vi "Write TIFF Metadata General.vi"(8 "error in (no error)":errorcluster, 10 "Destination Image Path":path=path "C:/Users/Sebastien/Desktop/TIFF/data_000000_Metadata.tif", 11 "Source File Image Path":path=path "C:/Users/Sebastien/Desktop/TIFF/data_000000.tif") -> (0 "Error Out":errorcluster)   [LabVIEW 2025]
doc: "This software was created to prototype writing metadata to a TIFF file with a single image.\n\n<B>Usage:</B> This software is free to use, copy or plagiariaze. It is provided \"as-is\", and no technical support will be provided. The copyright is retained by NASA Marshall Space Flight Center.\n\n<B>Testing:</B> This software was tested by A) verifying that operations were completed successfully using LabVIEW 2009 on Windows XP, .NET version 4.0 and B) Windows Vista Microsoft Office Picture Manager was able to read and display the output file and C) Windows Vista Windows Photo Gallery was able to read and display the output file and the Description and D) Adobe Photoshop for Macintosh was able to correctly load and display the image and all the metadata.\n\n<B>Note:</B> This software requires .NET version 4.0\n\n<B>Warning:</B> This software will overwrite the destination file if it exists.\n\nThis software originally developed by:\nDerek Mayer\nBAE Systems - Technology Solutions & Services\n308 Voyager Way\nHuntsville, AL 35806\n(256) 890-8000\nwww.mevatec.com\nwww.baesystems.com/TSS\nSeptember 2010"
uses:
  System.Drawing
panel:
  out "Metadata OUT":T1(array[cluster])
  out "Metadata":T2
  in  "Description":string="Embryo - GFP-Septin - RFP-Myosin"
  in  "User":T3(ring)
  # "https://forums.ni.com/t5/LabVIEW/How-do-I-add-meta-tag-data-to-a-TIF-image-file/td-p/1221780"
  # "https://exiv2.org/tags.html"
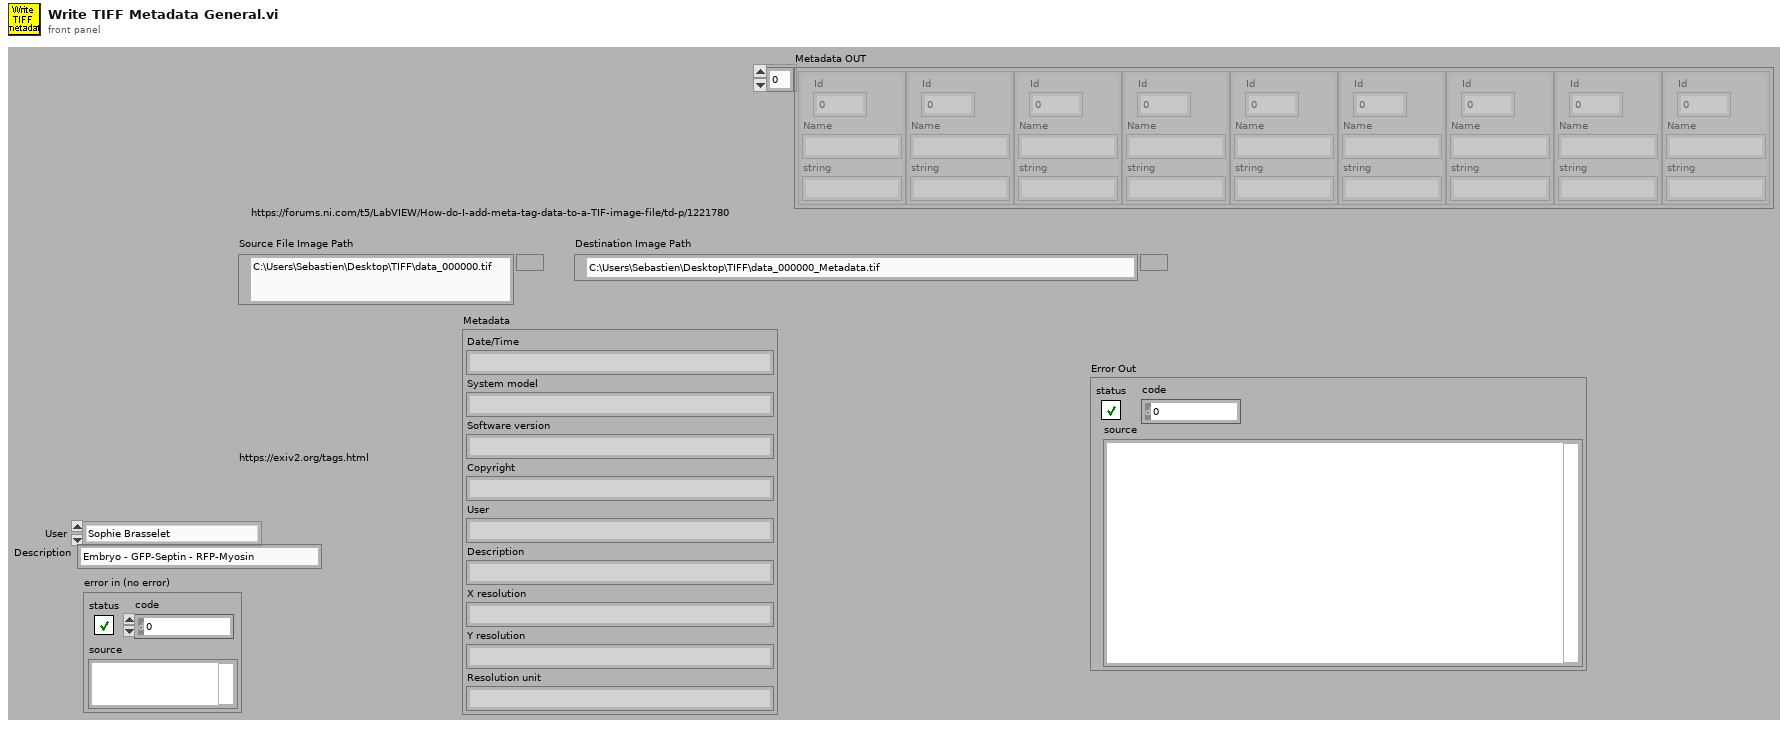
[diagram p1: front panel]
types:
  T1 = cluster{"Id":i32, "Name":string, "string":string}[]
  T2 = cluster{"Date/Time":string, "System model":string, "Software version":string, "Copyright":string, "User":string, "Description":string, "X resolution":string, "Y resolution":string, "Resolution unit":string}
  T3 = enum16{"Sophie Brasselet", "Jean-Jacques Honorine", "Sébastien Mailfert", "Manos Mavrakis"}
  T4 = cluster{"Error":errorcluster, "Source Filestream":refnum<k24>, "TIFF Decoder":refnum<k24>, "TIFF Frames":refnum<k24>, "get_Item":refnum<k24>, "Bitmap Metadata":refnum<k24>, "New Encoder":refnum<k24>}
  T5 = cluster{"ID":i32, "Name":string, "Notes":string}[]
  T6 = cluster{"Id":i32, "Name":string, "string":string}
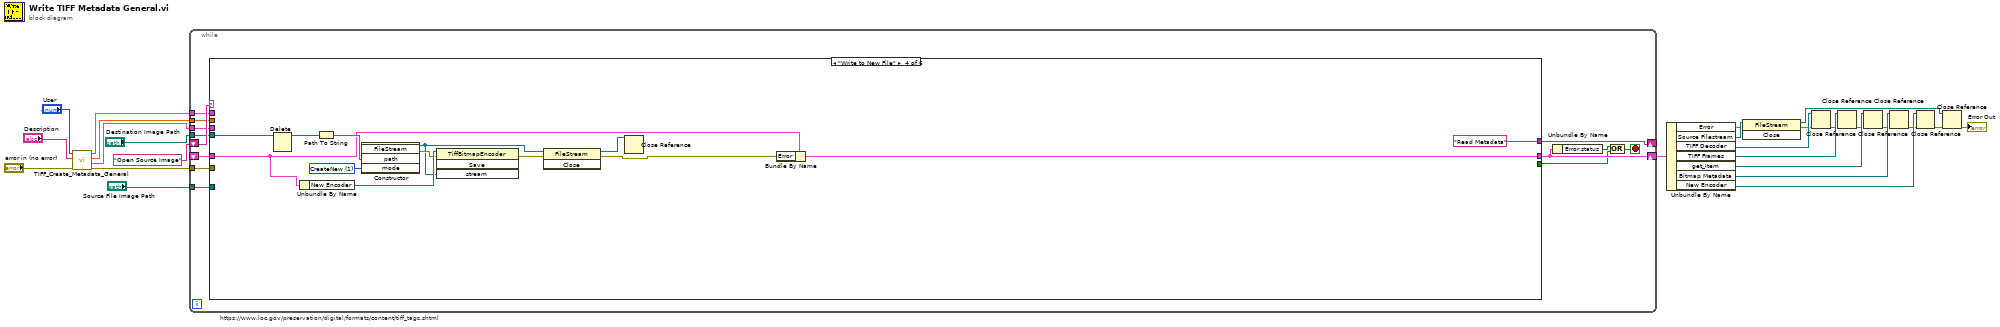
[diagram p0: block diagram]
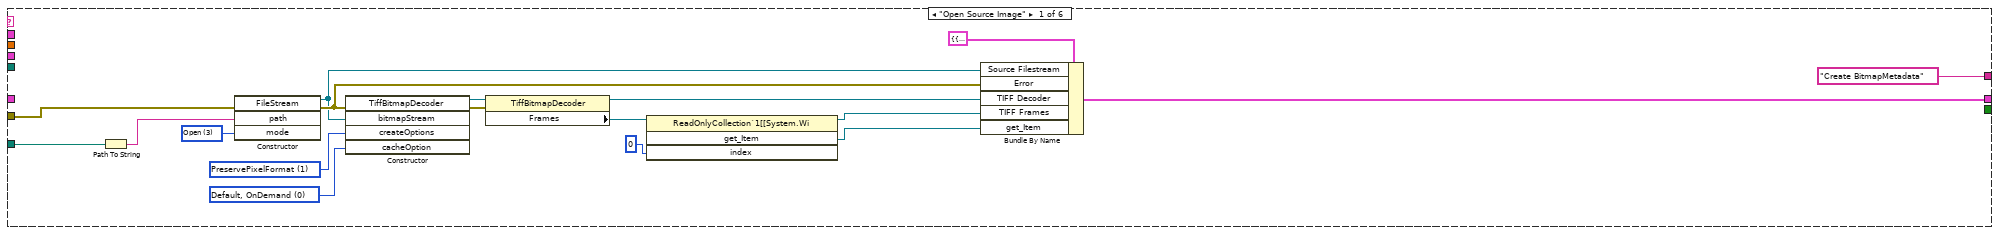
[diagram p2: hidden frame]
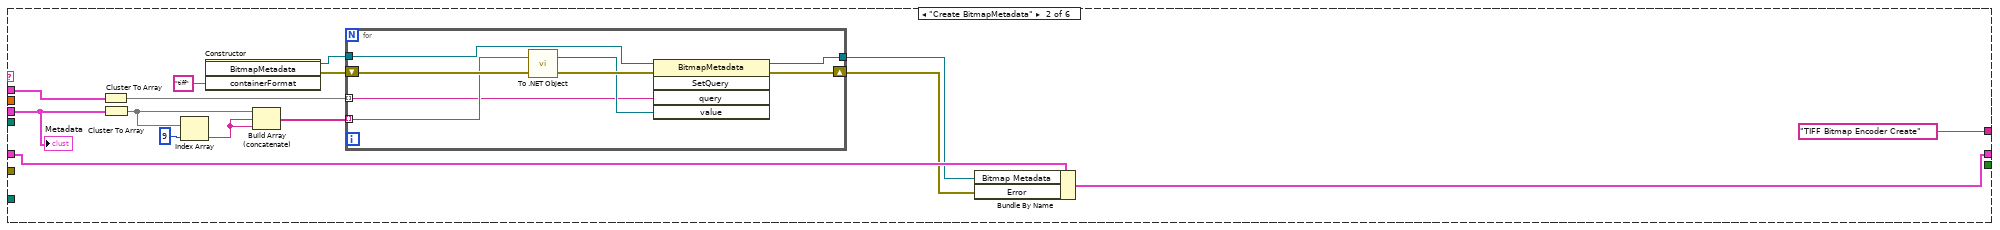
[diagram p3: hidden frame]
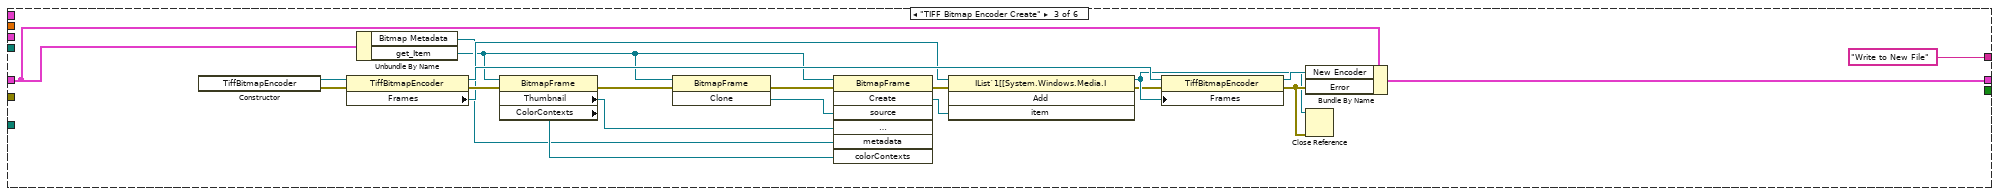
[diagram p4: hidden frame]
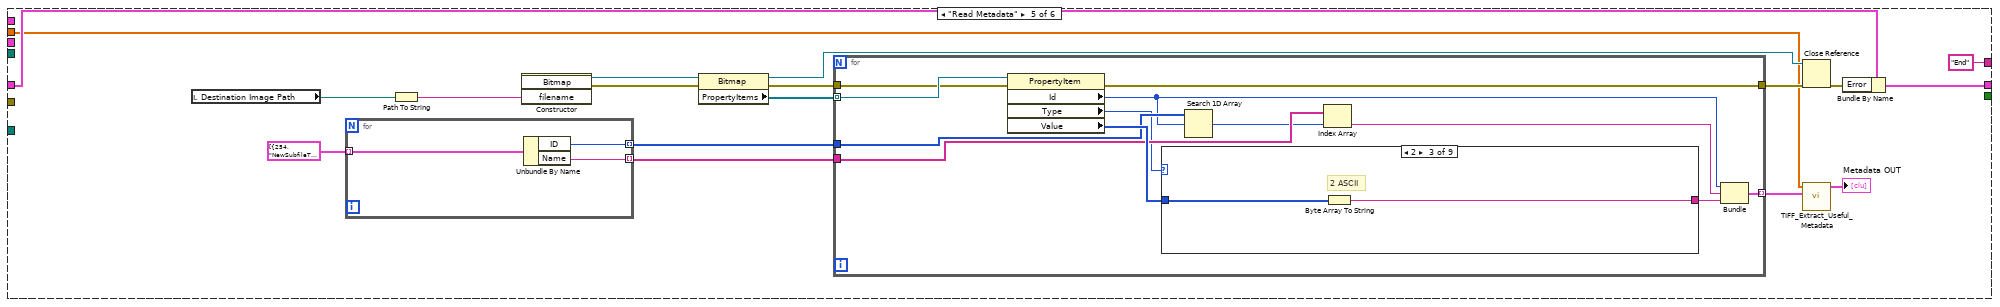
[diagram p5: hidden frame]
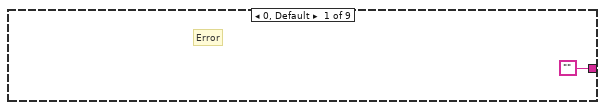
[diagram p6: hidden frame]
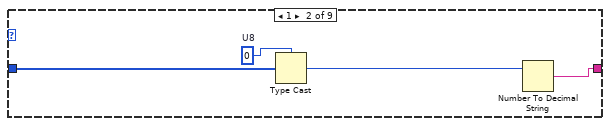
[diagram p7: hidden frame]
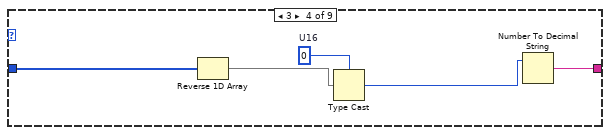
[diagram p8: hidden frame]
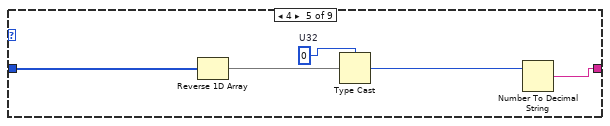
[diagram p9: hidden frame]
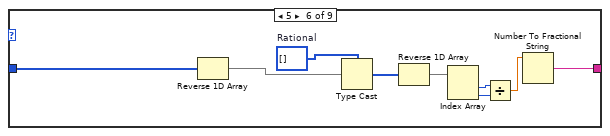
[diagram p10: hidden frame]
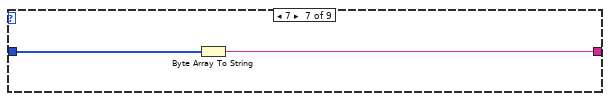
[diagram p11: hidden frame]
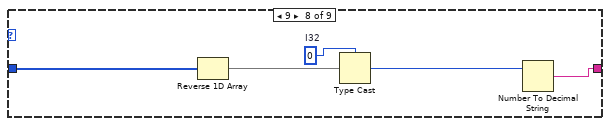
[diagram p12: hidden frame]
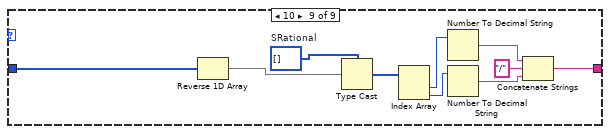
[diagram p13: hidden frame]
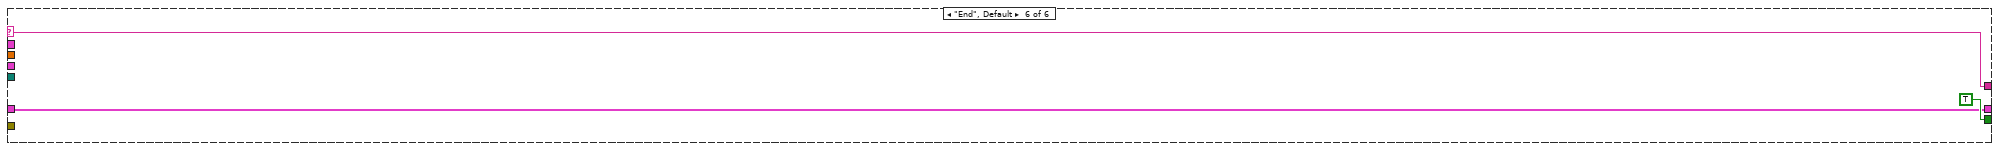
[diagram p14: hidden frame]
diagram:
  # "https://www.loc.gov/preservation/digital/formats/content/tiff_tags.shtml"
  n1 = call "TIFF_Create_Metadata_General.vi"("error in (no error)"="error in (no error)", "Description"="Description", "User"="User") -> ("error out"=w4:errorcluster, "Metadata OUT"=w2:T2, "Tag IDs"=w1:dbl[], "Taggs"=w3:T2)  [unwired: 5 in]
  n2 = while {
    shift-right: [w32] -> _
    shift-left: "Open Source Image" -> [w39]
    tunnel: "Source File Image Path" -> [w38]
    shift-right: [w37] -> w24
    shift-left: _ -> [w33]
    tunnel: "Destination Image Path" -> [w31]
    tunnel: w4 -> [w30]
    tunnel: w2 -> [w29]
    tunnel: w3 -> [w28]
    tunnel: w1 -> [w27]
    stop <- w34 stop-if-true
    n3 = case shown="\"Write to New File\"" w39 {
      selector: w39 -> [_ _ _ _ _ w191]
      tunnel: [_ _ _ _ _ TRUE] -> w36
      tunnel: w38 -> [w57 _ _ _ _ _]
      tunnel: [w53 w71 w101 w104 w119 w192] -> w37
      tunnel: w33 -> [_ w70 w98 w105 w120 w192]
      tunnel: ["Create BitmapMetadata" "TIFF Bitmap Encoder Create" "Write to New File" "Read Metadata" "End" w191] -> w32
      tunnel: w31 -> [_ _ _ w102 _ _]
      tunnel: w30 -> [w40 _ _ _ _ _]
      tunnel: w29 -> [_ w59 _ _ _ _]
      tunnel: w28 -> [_ w58 _ _ _ _]
      tunnel: w27 -> [_ _ _ _ w115 _]
      frame "Open Source Image" {
        w51 = 0 items=["Default, OnDemand", "OnLoad", "None"] ("cacheOption")
        w52 = 1 items=["None"=0, "PreservePixelFormat"=1, "DelayCreation"=2, "IgnoreColorProfile"=4, "IgnoreImageCache"=8] ("createOptions")
        w55 = 3 items=["CreateNew"=1, "Create"=2, "Open"=3, "OpenOrCreate"=4, "Truncate"=5, "Append"=6] ("mode")
        n4 = Path To String(path=w57) -> (string=w56:string)
        n5 = constructor class="FileStream"(error in=w40, "path"=w56, "mode"=w55) -> (reference out=w45:refnum<k24>, error out=w50:errorcluster)  [unwired: 2 in, 3 out]
        n6 = constructor class="TiffBitmapDecoder"(error in=w50, "bitmapStream"=w45, "createOptions"=w52, "cacheOption"=w51) -> (reference out=w48:refnum<k24>, error out=w49:errorcluster)  [unwired: 2 in, 4 out]
        n7 = property class="TiffBitmapDecoder"(reference=w48, error in=w49) -> (reference out=w44:refnum<k24>, "Frames"=w47:refnum<k24>)  [unwired: 1 out]
        n8 = invoke class="ReadOnlyCollection`1[[System.Wi" method="get_Item"(reference=w47, "index"=0) -> (reference out=w43:refnum<k24>, "get_Item"=w42:refnum<k24>)  [unwired: 2 in, 2 out]
        n9 = Bundle By Name(cluster=T4 {"Error"={"status"=FALSE, "code"=0, "source"=""}, "Source Filestream"=refnum, "TIFF Decoder"=refnum, "TIFF Frames"=refnum, "get_Item"=refnum, "Bitmap Metadata"=refnum, "New Encoder"=refnum}, "Source Filestream"=w45, "Error"=w50, "TIFF Decoder"=w44, "TIFF Frames"=w43, "get_Item"=w42) -> (w53:T4)
      }
      frame "Create BitmapMetadata" {
        n10 = Cluster To Array(cluster=w58) -> (array=w60:string[])
        n11 = Cluster To Array(cluster=w59) -> (array=w63:string[])
        n12 = Index Array(array=w63, index=9) -> (element=w64:string)
        n13 = constructor class="BitmapMetadata"("containerFormat"="tiff") -> (reference out=w69:refnum<k24>, error out=w68:errorcluster)  [unwired: 3 in, 2 out]
        n14 = Build Array (concatenate)(w63, w64, w64) -> (w62:string[])
        n15 = for {
          tunnel: [w77] -> w61
          tunnel: w69 -> [w74]
          shift-right: [w75] -> w66
          shift-left: w68 -> [w80]
          tunnel: w60 -> [w73] mode=indexing
          tunnel: w62 -> [w76] mode=indexing
          n16 = call <vilib>:"To .NET Object.vi"("error in (no error)"=w80, "anything"=w76) -> ("error out"=w79:errorcluster, ".NET object"=w78:refnum<k24>)
          n17 = invoke class="BitmapMetadata" method="SetQuery"(reference=w74, error in=w79, "query"=w73, "value"=w78) -> (reference out=w77:refnum<k24>, error out=w75:errorcluster)  [unwired: 1 in, 3 out]
        }
        n18 = Bundle By Name(cluster=w70, "Bitmap Metadata"=w61, "Error"=w66) -> (w71:T4)
        "Metadata" <- w59
      }
      frame "TIFF Bitmap Encoder Create" {
        n19 = constructor class="TiffBitmapEncoder"() -> (reference out=w90:refnum<k24>, error out=w99:errorcluster)  [unwired: 3 in, 1 out]
        n20 = property class="TiffBitmapEncoder"(reference=w90, error in=w99) -> (reference out=w94:refnum<k24>, error out=w93:errorcluster, "Frames"=w89:refnum<k24>)
        n21 = Unbundle By Name(w98) -> ("Bitmap Metadata"=w85:refnum<k24>, "get_Item"=w83:refnum<k24>)
        n22 = property class="BitmapFrame"(reference=w83, error in=w93) -> (error out=w95:errorcluster, "Thumbnail"=w87:refnum<k24>, "ColorContexts"=w88:refnum<k24>)  [unwired: 1 out]
        n23 = invoke class="BitmapFrame" method="Clone"(reference=w83, error in=w95) -> (error out=w82:errorcluster, "Clone"=w86:refnum<k24>)  [unwired: 1 in, 1 out]
        n24 = invoke class="BitmapFrame" method="Create"(reference=w83, error in=w82, "source"=w86, "thumbnail"=w87, "metadata"=w85, "colorContexts"=w88) -> (error out=w81:errorcluster, "Create"=w84:refnum<k24>)  [unwired: 1 in, 5 out]
        n25 = invoke class="IList`1[[System.Windows.Media.I" method="Add"(reference=w89, error in=w81, "item"=w84) -> (reference out=w92:refnum<k24>, error out=w91:errorcluster)  [unwired: 1 in, 2 out]
        n26 = property class="TiffBitmapEncoder"(reference=w94, error in=w91, "Frames"=w92) -> (reference out=w97:refnum<k24>, error out=w96:errorcluster)
        n27 = Bundle By Name(cluster=w98, "New Encoder"=w97, "Error"=w96) -> (w101:T4)
        n28 = Close Reference(reference=w92, error in (no error)=w96) -> ()  [unwired: 1 out]
      }
      frame "Write to New File" {
        w111 = 1 items=["CreateNew"=1, "Create"=2, "Open"=3, "OpenOrCreate"=4, "Truncate"=5, "Append"=6] ("mode")
        n29 = Delete(path (use dialog)=w102) -> (deleted path=w113:path)  [unwired: 4 in, 2 out]
        n30 = Unbundle By Name(w105) -> ("New Encoder"=w110:refnum<k24>)
        n31 = Path To String(path=w113) -> (string=w112:string)
        n32 = constructor class="FileStream"("path"=w112, "mode"=w111) -> (reference out=w108:refnum<k24>, error out=w109:errorcluster)  [unwired: 3 in, 3 out]
        n33 = invoke class="TiffBitmapEncoder" method="Save"(reference=w110, error in=w109, "stream"=w108) -> (error out=w107:errorcluster)  [unwired: 1 in, 3 out]
        n34 = invoke class="FileStream" method="Close"(reference=w108, error in=w107) -> (reference out=w103:refnum<k24>, error out=w106:errorcluster)  [unwired: 1 in, 1 out]
        n35 = Close Reference(reference=w103) -> ()  [unwired: 1 in, 1 out]
        n36 = Bundle By Name(cluster=w105, "Error"=w106) -> (w104:T4)
      }
      frame "Read Metadata" {
        n37 = local read "Destination Image Path"() -> (w122:path)
        n38 = for {
          tunnel: T5 [{"ID"=254, "Name"="NewSubfileType", "Notes"="A general indication of the kind of data contained in this subfile."}, {"ID"=255, "Name"="SubfileType", "Notes"="A general indication of the kind of data contained in this subfile."}, {"ID"=256, "Name"="ImageWidth", "Notes"="\"The number of columns in the image, i.e., the number of pixels per row.\""}, {"ID"=257, "Name"="ImageLength", "Notes"="The number of rows of pixels in the image."}, {"ID"=258, "Name"="BitsPerSample", "Notes"="Number of bits per component."}, {"ID"=259, "Name"="Compression", "Notes"="Compression scheme used on the image data."}, {"ID"=262, "Name"="PhotometricInterpretation", "Notes"="The color space of the image data."}, {"ID"=263, "Name"="Threshholding", "Notes"="\"For black and white TIFF files that represent shades of gray, the technique used to convert from gray to black and white pixels.\""}, {"ID"=264, "Name"="CellWidth", "Notes"="The width of the dithering or halftoning matrix used to create a dithered or halftoned bilevel file."}, {"ID"=265, "Name"="CellLength", "Notes"="The length of the dithering or halftoning matrix used to create a dithered or halftoned bilevel file."}, {"ID"=266, "Name"="FillOrder", "Notes"="The logical order of bits within a byte."}, {"ID"=269, "Name"="DocumentName", "Notes"="The name of the document from which this image was scanned."}, {"ID"=270, "Name"="ImageDescription", "Notes"="A string that describes the subject of the image."}, {"ID"=271, "Name"="Make", "Notes"="The scanner manufacturer."}, {"ID"=272, "Name"="Model", "Notes"="The scanner model name or number."}, {"ID"=273, "Name"="StripOffsets", "Notes"="\"For each strip, the byte offset of that strip.\""}, {"ID"=274, "Name"="Orientation", "Notes"="The orientation of the image with respect to the rows and columns."}, {"ID"=277, "Name"="SamplesPerPixel", "Notes"="The number of components per pixel."}, {"ID"=278, "Name"="RowsPerStrip", "Notes"="The number of rows per strip."}, {"ID"=279, "Name"="StripByteCounts", "Notes"="\"For each strip, the number of bytes in the strip after compression.\""}, {"ID"=280, "Name"="MinSampleValue", "Notes"="The minimum component value used."}, {"ID"=281, "Name"="MaxSampleValue", "Notes"="The maximum component value used."}, {"ID"=282, "Name"="XResolution", "Notes"="The number of pixels per ResolutionUnit in the ImageWidth direction."}, {"ID"=283, "Name"="YResolution", "Notes"="The number of pixels per ResolutionUnit in the ImageLength direction."}, {"ID"=284, "Name"="PlanarConfiguration", "Notes"="How the components of each pixel are stored."}, {"ID"=285, "Name"="PageName", "Notes"="The name of the page from which this image was scanned."}, {"ID"=286, "Name"="XPosition", "Notes"="X position of the image."}, {"ID"=287, "Name"="YPosition", "Notes"="Y position of the image."}, {"ID"=288, "Name"="FreeOffsets", "Notes"="\"For each string of contiguous unused bytes in a TIFF file, the byte offset of the string.\""}, {"ID"=289, "Name"="FreeByteCounts", "Notes"="\"For each string of contiguous unused bytes in a TIFF file, the number of bytes in the string.\""}, {"ID"=290, "Name"="GrayResponseUnit", "Notes"="The precision of the information contained in the GrayResponseCurve."}, {"ID"=291, "Name"="GrayResponseCurve", "Notes"="\"For grayscale data, the optical density of each possible pixel value.\""}, {"ID"=292, "Name"="T4Options", "Notes"="Options for Group 3 Fax compression"}, {"ID"=293, "Name"="T6Options", "Notes"="Options for Group 4 Fax compression"}, {"ID"=296, "Name"="ResolutionUnit", "Notes"="The unit of measurement for XResolution and YResolution."}, {"ID"=297, "Name"="PageNumber", "Notes"="The page number of the page from which this image was scanned."}, {"ID"=301, "Name"="TransferFunction", "Notes"="Describes a transfer function for the image in tabular style."}, {"ID"=305, "Name"="Software", "Notes"="Name and version number of the software package(s) used to create the image."}, {"ID"=306, "Name"="DateTime", "Notes"="Date and time of image creation."}, {"ID"=315, "Name"="Artist", "Notes"="Person who created the image."}, {"ID"=316, "Name"="HostComputer", "Notes"="The computer and/or operating system in use at the time of image creation."}, {"ID"=317, "Name"="Predictor", "Notes"="A mathematical operator that is applied to the image data before an encoding scheme is applied."}, {"ID"=318, "Name"="WhitePoint", "Notes"="The chromaticity of the white point of the image."}, {"ID"=319, "Name"="PrimaryChromaticities", "Notes"="The chromaticities of the primaries of the image."}, {"ID"=320, "Name"="ColorMap", "Notes"="A color map for palette color images."}, {"ID"=321, "Name"="HalftoneHints", "Notes"="Conveys to the halftone function the range of gray levels within a colorimetrically-specified image that should retain tonal detail."}, {"ID"=322, "Name"="TileWidth", "Notes"="The tile width in pixels. This is the number of columns in each tile."}, {"ID"=323, "Name"="TileLength", "Notes"="The tile length (height) in pixels. This is the number of rows in each tile."}, {"ID"=324, "Name"="TileOffsets", "Notes"="\"For each tile, the byte offset of that tile, as compressed and stored on disk.\""}, {"ID"=325, "Name"="TileByteCounts", "Notes"="\"For each tile, the number of (compressed) bytes in that tile.\""}, {"ID"=326, "Name"="BadFaxLines", "Notes"="\"Used in the TIFF-F standard, denotes the number of 'bad' scan lines encountered by the facsimile device.\""}, {"ID"=327, "Name"="CleanFaxData", "Notes"="\"Used in the TIFF-F standard, indicates if 'bad' lines encountered during reception are stored in the data, or if 'bad' lines have been replaced by the receiver.\""}, {"ID"=328, "Name"="ConsecutiveBadFaxLines", "Notes"="\"Used in the TIFF-F standard, denotes the maximum number of consecutive 'bad' scanlines received.\""}, {"ID"=330, "Name"="SubIFDs", "Notes"="Offset to child IFDs."}, {"ID"=332, "Name"="InkSet", "Notes"="The set of inks used in a separated (PhotometricInterpretation=5) image."}, {"ID"=333, "Name"="InkNames", "Notes"="The name of each ink used in a separated image."}, {"ID"=334, "Name"="NumberOfInks", "Notes"="The number of inks."}, {"ID"=336, "Name"="DotRange", "Notes"="The component values that correspond to a 0% dot and 100% dot."}, {"ID"=337, "Name"="TargetPrinter", "Notes"="A description of the printing environment for which this separation is intended."}, {"ID"=338, "Name"="ExtraSamples", "Notes"="Description of extra components."}, {"ID"=339, "Name"="SampleFormat", "Notes"="Specifies how to interpret each data sample in a pixel."}, {"ID"=340, "Name"="SMinSampleValue", "Notes"="Specifies the minimum sample value."}, {"ID"=341, "Name"="SMaxSampleValue", "Notes"="Specifies the maximum sample value."}, {"ID"=342, "Name"="TransferRange", "Notes"="Expands the range of the TransferFunction."}, {"ID"=343, "Name"="ClipPath", "Notes"="Mirrors the essentials of PostScript's path creation functionality."}, {"ID"=344, "Name"="XClipPathUnits", "Notes"="\"The number of units that span the width of the image, in terms of integer ClipPath coordinates.\""}, {"ID"=345, "Name"="YClipPathUnits", "Notes"="\"The number of units that span the height of the image, in terms of integer ClipPath coordinates.\""}, {"ID"=346, "Name"="Indexed", "Notes"="Aims to broaden the support for indexed images to include support for any color space."}, {"ID"=347, "Name"="JPEGTables", "Notes"="JPEG quantization and/or Huffman tables."}, {"ID"=351, "Name"="OPIProxy", "Notes"="OPI-related."}, {"ID"=400, "Name"="GlobalParametersIFD", "Notes"="Used in the TIFF-FX standard to point to an IFD containing tags that are globally applicable to the complete TIFF file."}, {"ID"=401, "Name"="ProfileType", "Notes"="\"Used in the TIFF-FX standard, denotes the type of data stored in this file or IFD.\""}, {"ID"=402, "Name"="FaxProfile", "Notes"="\"Used in the TIFF-FX standard, denotes the 'profile' that applies to this file.\""}, {"ID"=403, "Name"="CodingMethods", "Notes"="\"Used in the TIFF-FX standard, indicates which coding methods are used in the file.\""}, {"ID"=404, "Name"="VersionYear", "Notes"="\"Used in the TIFF-FX standard, denotes the year of the standard specified by the FaxProfile field.\""}, {"ID"=405, "Name"="ModeNumber", "Notes"="\"Used in the TIFF-FX standard, denotes the mode of the standard specified by the FaxProfile field.\""}, {"ID"=433, "Name"="Decode", "Notes"="\"Used in the TIFF-F and TIFF-FX standards, holds information about the ITULAB (PhotometricInterpretation = 10) encoding.\""}, {"ID"=434, "Name"="DefaultImageColor", "Notes"="\"Defined in the Mixed Raster Content part of RFC 2301, is the default color needed in areas where no image is available.\""}, {"ID"=512, "Name"="JPEGProc", "Notes"="Old-style JPEG compression field. TechNote2 invalidates this part of the specification."}, {"ID"=513, "Name"="JPEGInterchangeFormat", "Notes"="Old-style JPEG compression field. TechNote2 invalidates this part of the specification."}, {"ID"=514, "Name"="JPEGInterchangeFormatLength", "Notes"="Old-style JPEG compression field. TechNote2 invalidates this part of the specification."}, {"ID"=515, "Name"="JPEGRestartInterval", "Notes"="Old-style JPEG compression field. TechNote2 invalidates this part of the specification."}, {"ID"=517, "Name"="JPEGLosslessPredictors", "Notes"="Old-style JPEG compression field. TechNote2 invalidates this part of the specification."}, {"ID"=518, "Name"="JPEGPointTransforms", "Notes"="Old-style JPEG compression field. TechNote2 invalidates this part of the specification."}, {"ID"=519, "Name"="JPEGQTables", "Notes"="Old-style JPEG compression field. TechNote2 invalidates this part of the specification."}, {"ID"=520, "Name"="JPEGDCTables", "Notes"="Old-style JPEG compression field. TechNote2 invalidates this part of the specification."}, {"ID"=521, "Name"="JPEGACTables", "Notes"="Old-style JPEG compression field. TechNote2 invalidates this part of the specification."}, {"ID"=529, "Name"="YCbCrCoefficients", "Notes"="The transformation from RGB to YCbCr image data."}, {"ID"=530, "Name"="YCbCrSubSampling", "Notes"="Specifies the subsampling factors used for the chrominance components of a YCbCr image."}, {"ID"=531, "Name"="YCbCrPositioning", "Notes"="Specifies the positioning of subsampled chrominance components relative to luminance samples."}, {"ID"=532, "Name"="ReferenceBlackWhite", "Notes"="Specifies a pair of headroom and footroom image data values (codes) for each pixel component."}, {"ID"=559, "Name"="StripRowCounts", "Notes"="\"Defined in the Mixed Raster Content part of RFC 2301, used to replace RowsPerStrip for IFDs with variable-sized strips.\""}, {"ID"=700, "Name"="XMP", "Notes"="XML packet containing XMP metadata"}, {"ID"=32781, "Name"="ImageID", "Notes"="OPI-related."}, {"ID"=32932, "Name"="Wang Annotation", "Notes"="\"Annotation data, as used in 'Imaging for Windows'.\""}, {"ID"=33432, "Name"="Copyright", "Notes"="Copyright notice."}, {"ID"=33434, "Name"="ExposureTime", "Notes"="\"Exposure time, given in seconds.\""}, {"ID"=33437, "Name"="FNumber", "Notes"="The F number."}, {"ID"=33445, "Name"="MD FileTag", "Notes"="Specifies the pixel data format encoding in the Molecular Dynamics GEL file format."}, {"ID"=33446, "Name"="MD ScalePixel", "Notes"="Specifies a scale factor in the Molecular Dynamics GEL file format."}, {"ID"=33447, "Name"="MD ColorTable", "Notes"="Used to specify the conversion from 16bit to 8bit in the Molecular Dynamics GEL file format."}, {"ID"=33448, "Name"="MD LabName", "Notes"="\"Name of the lab that scanned this file, as used in the Molecular Dynamics GEL file format.\""}, {"ID"=33449, "Name"="MD SampleInfo", "Notes"="\"Information about the sample, as used in the Molecular Dynamics GEL file format.\""}, {"ID"=33450, "Name"="MD PrepDate", "Notes"="\"Date the sample was prepared, as used in the Molecular Dynamics GEL file format.\""}, {"ID"=33451, "Name"="MD PrepTime", "Notes"="\"Time the sample was prepared, as used in the Molecular Dynamics GEL file format.\""}, {"ID"=33452, "Name"="MD FileUnits", "Notes"="\"Units for data in this file, as used in the Molecular Dynamics GEL file format.\""}, {"ID"=33550, "Name"="ModelPixelScaleTag", "Notes"="Used in interchangeable GeoTIFF files."}, {"ID"=33723, "Name"="IPTC", "Notes"="IPTC (International Press Telecommunications Council) metadata."}, {"ID"=33918, "Name"="INGR Packet Data Tag", "Notes"="Intergraph Application specific storage."}, {"ID"=33919, "Name"="INGR Flag Registers", "Notes"="Intergraph Application specific flags."}, {"ID"=33920, "Name"="IrasB Transformation Matrix", "Notes"="\"Originally part of Intergraph's GeoTIFF tags, but likely understood by IrasB only.\""}, {"ID"=33922, "Name"="ModelTiepointTag", "Notes"="\"Originally part of Intergraph's GeoTIFF tags, but now used in interchangeable GeoTIFF files.\""}, {"ID"=34264, "Name"="ModelTransformationTag", "Notes"="Used in interchangeable GeoTIFF files."}, {"ID"=34377, "Name"="Photoshop", "Notes"="Collection of Photoshop 'Image Resource Blocks'."}, {"ID"=34665, "Name"="Exif IFD", "Notes"="A pointer to the Exif IFD."}, {"ID"=34675, "Name"="ICC Profile", "Notes"="ICC profile data."}, {"ID"=34732, "Name"="ImageLayer", "Notes"="\"Defined in the Mixed Raster Content part of RFC 2301, used to denote the particular function of this Image in the mixed raster scheme.\""}, {"ID"=34735, "Name"="GeoKeyDirectoryTag", "Notes"="Used in interchangeable GeoTIFF files."}, {"ID"=34736, "Name"="GeoDoubleParamsTag", "Notes"="Used in interchangeable GeoTIFF files."}, {"ID"=34737, "Name"="GeoAsciiParamsTag", "Notes"="Used in interchangeable GeoTIFF files."}, {"ID"=34850, "Name"="ExposureProgram", "Notes"="The class of the program used by the camera to set exposure when the picture is taken."}, {"ID"=34852, "Name"="SpectralSensitivity", "Notes"="Indicates the spectral sensitivity of each channel of the camera used."}, {"ID"=34853, "Name"="GPS IFD", "Notes"="A pointer to the Exif-related GPS Info IFD."}, {"ID"=34855, "Name"="ISOSpeedRatings", "Notes"="Indicates the ISO Speed and ISO Latitude of the camera or input device as specified in ISO 12232."}, {"ID"=34856, "Name"="OECF", "Notes"="Indicates the Opto-Electric Conversion Function (OECF) specified in ISO 14524."}, {"ID"=34908, "Name"="HylaFAX FaxRecvParams", "Notes"="Used by HylaFAX."}, {"ID"=34909, "Name"="HylaFAX FaxSubAddress", "Notes"="Used by HylaFAX."}, {"ID"=34910, "Name"="HylaFAX FaxRecvTime", "Notes"="Used by HylaFAX."}, {"ID"=36864, "Name"="ExifVersion", "Notes"="The version of the supported Exif standard."}, {"ID"=36867, "Name"="DateTimeOriginal", "Notes"="The date and time when the original image data was generated."}, {"ID"=36868, "Name"="DateTimeDigitized", "Notes"="The date and time when the image was stored as digital data."}, {"ID"=37121, "Name"="ComponentsConfiguration", "Notes"="Specific to compressed data; specifies the channels and complements PhotometricInterpretation"}, {"ID"=37122, "Name"="CompressedBitsPerPixel", "Notes"="Specific to compressed data; states the compressed bits per pixel."}, {"ID"=37377, "Name"="ShutterSpeedValue", "Notes"="Shutter speed."}, {"ID"=37378, "Name"="ApertureValue", "Notes"="The lens aperture."}, {"ID"=37379, "Name"="BrightnessValue", "Notes"="The value of brightness."}, {"ID"=37380, "Name"="ExposureBiasValue", "Notes"="The exposure bias."}, {"ID"=37381, "Name"="MaxApertureValue", "Notes"="The smallest F number of the lens."}, {"ID"=37382, "Name"="SubjectDistance", "Notes"="\"The distance to the subject, given in meters.\""}, {"ID"=37383, "Name"="MeteringMode", "Notes"="The metering mode."}, {"ID"=37384, "Name"="LightSource", "Notes"="The kind of light source."}, {"ID"=37385, "Name"="Flash", "Notes"="Indicates the status of flash when the image was shot."}, {"ID"=37386, "Name"="FocalLength", "Notes"="\"The actual focal length of the lens, in mm.\""}, {"ID"=37396, "Name"="SubjectArea", "Notes"="Indicates the location and area of the main subject in the overall scene."}, {"ID"=37500, "Name"="MakerNote", "Notes"="Manufacturer specific information."}, {"ID"=37510, "Name"="UserComment", "Notes"="Keywords or comments on the image; complements ImageDescription."}, {"ID"=37520, "Name"="SubsecTime", "Notes"="A tag used to record fractions of seconds for the DateTime tag."}, {"ID"=37521, "Name"="SubsecTimeOriginal", "Notes"="A tag used to record fractions of seconds for the DateTimeOriginal tag."}, {"ID"=37522, "Name"="SubsecTimeDigitized", "Notes"="A tag used to record fractions of seconds for the DateTimeDigitized tag."}, {"ID"=37724, "Name"="ImageSourceData", "Notes"="Used by Adobe Photoshop."}, {"ID"=40960, "Name"="FlashpixVersion", "Notes"="The Flashpix format version supported by a FPXR file."}, {"ID"=40961, "Name"="ColorSpace", "Notes"="The color space information tag is always recorded as the color space specifier."}, {"ID"=40962, "Name"="PixelXDimension", "Notes"="Specific to compressed data; the valid width of the meaningful image."}, {"ID"=40963, "Name"="PixelYDimension", "Notes"="Specific to compressed data; the valid height of the meaningful image."}, {"ID"=40964, "Name"="RelatedSoundFile", "Notes"="Used to record the name of an audio file related to the image data."}, {"ID"=40965, "Name"="Interoperability IFD", "Notes"="A pointer to the Exif-related Interoperability IFD."}, {"ID"=41483, "Name"="FlashEnergy", "Notes"="\"Indicates the strobe energy at the time the image is captured, as measured in Beam Candle Power Seconds\""}, {"ID"=41484, "Name"="SpatialFrequencyResponse", "Notes"="\"Records the camera or input device spatial frequency table and SFR values in the direction of image width, image height, and diagonal direction, as specified in ISO 12233.\""}, {"ID"=41486, "Name"="FocalPlaneXResolution", "Notes"="Indicates the number of pixels in the image width (X) direction per FocalPlaneResolutionUnit on the camera focal plane."}, {"ID"=41487, "Name"="FocalPlaneYResolution", "Notes"="Indicates the number of pixels in the image height (Y) direction per FocalPlaneResolutionUnit on the camera focal plane."}, {"ID"=41488, "Name"="FocalPlaneResolutionUnit", "Notes"="Indicates the unit for measuring FocalPlaneXResolution and FocalPlaneYResolution."}, {"ID"=41492, "Name"="SubjectLocation", "Notes"="Indicates the location of the main subject in the scene."}, {"ID"=41493, "Name"="ExposureIndex", "Notes"="Indicates the exposure index selected on the camera or input device at the time the image is captured."}, {"ID"=41495, "Name"="SensingMethod", "Notes"="Indicates the image sensor type on the camera or input device."}, {"ID"=41728, "Name"="FileSource", "Notes"="Indicates the image source."}, {"ID"=41729, "Name"="SceneType", "Notes"="Indicates the type of scene."}, {"ID"=41730, "Name"="CFAPattern", "Notes"="Indicates the color filter array (CFA) geometric pattern of the image sensor when a one-chip color area sensor is used."}, {"ID"=41985, "Name"="CustomRendered", "Notes"="\"Indicates the use of special processing on image data, such as rendering geared to output.\""}, {"ID"=41986, "Name"="ExposureMode", "Notes"="Indicates the exposure mode set when the image was shot."}, {"ID"=41987, "Name"="WhiteBalance", "Notes"="Indicates the white balance mode set when the image was shot."}, {"ID"=41988, "Name"="DigitalZoomRatio", "Notes"="Indicates the digital zoom ratio when the image was shot."}, {"ID"=41989, "Name"="FocalLengthIn35mmFilm", "Notes"="\"Indicates the equivalent focal length assuming a 35mm film camera, in mm.\""}, {"ID"=41990, "Name"="SceneCaptureType", "Notes"="Indicates the type of scene that was shot."}, {"ID"=41991, "Name"="GainControl", "Notes"="Indicates the degree of overall image gain adjustment."}, {"ID"=41992, "Name"="Contrast", "Notes"="Indicates the direction of contrast processing applied by the camera when the image was shot."}, {"ID"=41993, "Name"="Saturation", "Notes"="Indicates the direction of saturation processing applied by the camera when the image was shot."}, {"ID"=41994, "Name"="Sharpness", "Notes"="Indicates the direction of sharpness processing applied by the camera when the image was shot."}, {"ID"=41995, "Name"="DeviceSettingDescription", "Notes"="This tag indicates information on the picture-taking conditions of a particular camera model."}, {"ID"=41996, "Name"="SubjectDistanceRange", "Notes"="Indicates the distance to the subject."}, {"ID"=42016, "Name"="ImageUniqueID", "Notes"="Indicates an identifier assigned uniquely to each image."}, {"ID"=42112, "Name"="GDAL_METADATA", "Notes"="\"Used by the GDAL library, holds an XML list of name=value 'metadata' values about the image as a whole, and about specific samples.\""}, {"ID"=42113, "Name"="GDAL_NODATA", "Notes"="\"Used by the GDAL library, contains an ASCII encoded nodata or background pixel value.\""}, {"ID"=50215, "Name"="Oce Scanjob Description", "Notes"="Used in the Oce scanning process."}, {"ID"=50216, "Name"="Oce Application Selector", "Notes"="Used in the Oce scanning process."}, {"ID"=50217, "Name"="Oce Identification Number", "Notes"="Used in the Oce scanning process."}, {"ID"=50218, "Name"="Oce ImageLogic Characteristics", "Notes"="Used in the Oce scanning process."}, {"ID"=50706, "Name"="DNGVersion", "Notes"="Used in IFD 0 of DNG files."}, {"ID"=50707, "Name"="DNGBackwardVersion", "Notes"="Used in IFD 0 of DNG files."}, {"ID"=50708, "Name"="UniqueCameraModel", "Notes"="Used in IFD 0 of DNG files."}, {"ID"=50709, "Name"="LocalizedCameraModel", "Notes"="Used in IFD 0 of DNG files."}, {"ID"=50710, "Name"="CFAPlaneColor", "Notes"="Used in Raw IFD of DNG files."}, {"ID"=50711, "Name"="CFALayout", "Notes"="Used in Raw IFD of DNG files."}, {"ID"=50712, "Name"="LinearizationTable", "Notes"="Used in Raw IFD of DNG files."}, {"ID"=50713, "Name"="BlackLevelRepeatDim", "Notes"="Used in Raw IFD of DNG files."}, {"ID"=50714, "Name"="BlackLevel", "Notes"="Used in Raw IFD of DNG files."}, {"ID"=50715, "Name"="BlackLevelDeltaH", "Notes"="Used in Raw IFD of DNG files."}, {"ID"=50716, "Name"="BlackLevelDeltaV", "Notes"="Used in Raw IFD of DNG files."}, {"ID"=50717, "Name"="WhiteLevel", "Notes"="Used in Raw IFD of DNG files."}, {"ID"=50718, "Name"="DefaultScale", "Notes"="Used in Raw IFD of DNG files."}, {"ID"=50719, "Name"="DefaultCropOrigin", "Notes"="Used in Raw IFD of DNG files."}, {"ID"=50720, "Name"="DefaultCropSize", "Notes"="Used in Raw IFD of DNG files."}, {"ID"=50721, "Name"="ColorMatrix1", "Notes"="Used in IFD 0 of DNG files."}, {"ID"=50722, "Name"="ColorMatrix2", "Notes"="Used in IFD 0 of DNG files."}, {"ID"=50723, "Name"="CameraCalibration1", "Notes"="Used in IFD 0 of DNG files."}, {"ID"=50724, "Name"="CameraCalibration2", "Notes"="Used in IFD 0 of DNG files."}, {"ID"=50725, "Name"="ReductionMatrix1", "Notes"="Used in IFD 0 of DNG files."}, {"ID"=50726, "Name"="ReductionMatrix2", "Notes"="Used in IFD 0 of DNG files."}, {"ID"=50727, "Name"="AnalogBalance", "Notes"="Used in IFD 0 of DNG files."}, {"ID"=50728, "Name"="AsShotNeutral", "Notes"="Used in IFD 0 of DNG files."}, {"ID"=50729, "Name"="AsShotWhiteXY", "Notes"="Used in IFD 0 of DNG files."}, {"ID"=50730, "Name"="BaselineExposure", "Notes"="Used in IFD 0 of DNG files."}, {"ID"=50731, "Name"="BaselineNoise", "Notes"="Used in IFD 0 of DNG files."}, {"ID"=50732, "Name"="BaselineSharpness", "Notes"="Used in IFD 0 of DNG files."}, {"ID"=50733, "Name"="BayerGreenSplit", "Notes"="Used in Raw IFD of DNG files."}, {"ID"=50734, "Name"="LinearResponseLimit", "Notes"="Used in IFD 0 of DNG files."}, {"ID"=50735, "Name"="CameraSerialNumber", "Notes"="Used in IFD 0 of DNG files."}, {"ID"=50736, "Name"="LensInfo", "Notes"="Used in IFD 0 of DNG files."}, {"ID"=50737, "Name"="ChromaBlurRadius", "Notes"="Used in Raw IFD of DNG files."}, {"ID"=50738, "Name"="AntiAliasStrength", "Notes"="Used in Raw IFD of DNG files."}, {"ID"=50740, "Name"="DNGPrivateData", "Notes"="Used in IFD 0 of DNG files."}, {"ID"=50741, "Name"="MakerNoteSafety", "Notes"="Used in IFD 0 of DNG files."}, {"ID"=50778, "Name"="CalibrationIlluminant1", "Notes"="Used in IFD 0 of DNG files."}, {"ID"=50779, "Name"="CalibrationIlluminant2", "Notes"="Used in IFD 0 of DNG files."}, {"ID"=50780, "Name"="BestQualityScale", "Notes"="Used in Raw IFD of DNG files."}, {"ID"=50784, "Name"="Alias Layer Metadata", "Notes"="Alias Sketchbook Pro layer usage description."}] ("EXIF Data list") -> [w135] mode=indexing
          tunnel: [w134] -> w129 mode=indexing
          tunnel: [w133] -> w130 mode=indexing
          n39 = Unbundle By Name(w135) -> ("ID"=w134:i32, "Name"=w133:string)
        }
        n40 = Path To String(path=w122) -> (string=w132:string)
        n41 = constructor class="Bitmap"("filename"=w132) -> (reference out=w128:refnum<k24>, error out=w127:errorcluster)  [unwired: 3 in, 2 out]
        n42 = property class="Bitmap"(reference=w128, error in=w127) -> (reference out=w126:refnum<k24>, error out=w125:errorcluster, "PropertyItems"=w124:refnum<k24>[])
        n43 = for {
          tunnel: w124 -> [w147] mode=indexing
          tunnel: [w146] -> w123
          tunnel: [w145] -> w117 mode=indexing
          tunnel: w129 -> [w141]
          tunnel: w130 -> [w139]
          tunnel: w125 -> [w144]
          n44 = property class="PropertyItem"(reference=w147, error in=w144) -> (error out=w146:errorcluster, "Id"=w140:i32, "Type"=w136:i16, "Value"=w143:u8[])  [unwired: 1 out]
          n45 = case shown="2" w136 {
            tunnel: w143 -> [_ w152 w154 w159 w164 w173 w175 w180 w190]
            tunnel: ["" w149 w153 w156 w161 w167 w174 w178 w184] -> w142
            frame 0, Default {
              # "Error"
            }
            frame 1 {
              w151 = u8 0  # U8
              n46 = Type Cast(type=w151, x=w152) -> (*(type *) &x=w150:u8)
              n47 = Number To Decimal String(number=w150) -> (decimal integer string=w149:string)  [unwired: 1 in]
            }
            frame 2 {
              # "2 ASCII"
              n48 = Byte Array To String(unsigned byte array=w154) -> (string=w153:string)
            }
            frame 3 {
              w157 = u16 0  # U16
              n49 = Reverse 1D Array(array=w159) -> (reversed array=w155:u8[])
              n50 = Type Cast(type=w157, x=w155) -> (*(type *) &x=w158:u16)
              n51 = Number To Decimal String(number=w158) -> (decimal integer string=w156:string)  [unwired: 1 in]
            }
            frame 4 {
              w162 = u32 0  # U32
              n52 = Reverse 1D Array(array=w164) -> (reversed array=w160:u8[])
              n53 = Type Cast(type=w162, x=w160) -> (*(type *) &x=w163:u32)
              n54 = Number To Decimal String(number=w163) -> (decimal integer string=w161:string)  [unwired: 1 in]
            }
            frame 5 {
              w172 = u32[] []  # Rational
              n55 = Reverse 1D Array(array=w173) -> (reversed array=w166:u8[])
              n56 = Type Cast(type=w172, x=w166) -> (*(type *) &x=w171:u32[])
              n57 = Reverse 1D Array(array=w171) -> (reversed array=w165:u32[])
              n58 = Index Array(array=w165) -> (element #1=w170:u32, element #2=w169:u32)  [unwired: 2 in]
              n59 = Divide(x=w170, y=w169) -> (x/y=w168:dbl)
              n60 = Number To Fractional String(number=w168) -> (F-format string=w167:string)  [unwired: 3 in]
            }
            frame 7 {
              n61 = Byte Array To String(unsigned byte array=w175) -> (string=w174:string)
            }
            frame 9 {
              w177 = 0  # I32
              n62 = Reverse 1D Array(array=w180) -> (reversed array=w176:u8[])
              n63 = Type Cast(type=w177, x=w176) -> (*(type *) &x=w179:i32)
              n64 = Number To Decimal String(number=w179) -> (decimal integer string=w178:string)  [unwired: 1 in]
            }
            frame 10 {
              w182 = i32[] []  # SRational
              n65 = Reverse 1D Array(array=w190) -> (reversed array=w181:u8[])
              n66 = Type Cast(type=w182, x=w181) -> (*(type *) &x=w189:i32[])
              n67 = Index Array(array=w189) -> (element #1=w187:i32, element #2=w188:i32)  [unwired: 2 in]
              n68 = Number To Decimal String(number=w187) -> (decimal integer string=w186:string)  [unwired: 1 in]
              n69 = Number To Decimal String(number=w188) -> (decimal integer string=w185:string)  [unwired: 1 in]
              n70 = Concatenate Strings(w186, "/" ("string"), w185) -> (w184:string)
            }
          }
          n71 = Search 1D Array(1D array=w141, element=w140) -> (index of element=w138:i32)  [unwired: 1 in]
          n72 = Index Array(array=w139, index=w138) -> (element=w137:string)
          n73 = Bundle("Id"=w140, "Name"=w137, "string"=w142) -> (w145:T6)  [unwired: 1 in]
        }
        n74 = Close Reference(reference=w126, error in (no error)=w123) -> (error out=w118:errorcluster)
        n75 = call "TIFF_Extract_Useful_Metadata.vi"("Array of Metadata IN"=w117, "Tag IDs"=w115) -> ("Array of useful Meatadata OUT"=→"Metadata OUT":T1)  [unwired: 9 in]
        n76 = Bundle By Name(cluster=w120, "Error"=w118) -> (w119:T4)
      }
      frame "End", Default {
      }
    }
    n77 = Unbundle By Name(w37) -> ("Error.status"=w35:bool)
    n78 = Compound Arithmetic op=OR(w35, w36) -> (w34:bool)
  }
  n79 = Unbundle By Name(w24) -> ("Error"=w15:errorcluster, "Source Filestream"=w17:refnum<k24>, "TIFF Decoder"=w23:refnum<k24>, "TIFF Frames"=w22:refnum<k24>, "get_Item"=w21:refnum<k24>, "Bitmap Metadata"=w20:refnum<k24>, "New Encoder"=w19:refnum<k24>)
  n80 = invoke class="FileStream" method="Close"(reference=w17, error in=w15) -> (reference out=w16:refnum<k24>, error out=w13:errorcluster)  [unwired: 1 in, 1 out]
  n81 = Close Reference(reference=w23, error in (no error)=w13) -> (error out=w12:errorcluster)
  n82 = Close Reference(reference=w22, error in (no error)=w12) -> (error out=w11:errorcluster)
  n83 = Close Reference(reference=w21, error in (no error)=w11) -> (error out=w10:errorcluster)
  n84 = Close Reference(reference=w20, error in (no error)=w10) -> (error out=w9:errorcluster)
  n85 = Close Reference(reference=w19, error in (no error)=w9) -> (error out=w8:errorcluster)
  n86 = Close Reference(reference=w16, error in (no error)=w8) -> (error out=→"Error Out":errorcluster)
